vi "test prepared statement.vi"() -> ()   [LabVIEW 2020, in "mysql.lvlib" / "mysql.lvclass"]
uses:
  mysql.net/mysql.lvclass
panel:
  in  "Connection string":string="server=127.0.0.1;uid=root;pwd=Nitrog3n;database=test"
  in  "error in (no error)":errorcluster
  out "mysql out":refnum<class "mysql.lvclass">
  out "error out":errorcluster
  in  "Statement in":string
  in  "Parameters in":string[](array[string])
  out "Result":string[][](array[string])
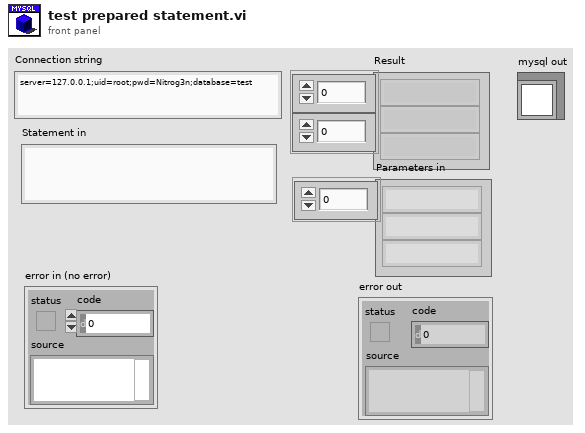
[diagram p1: front panel]
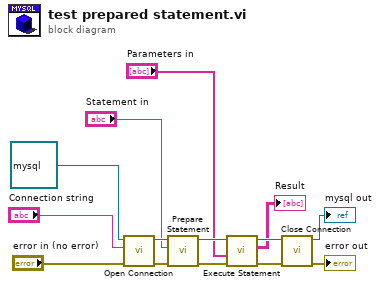
[diagram p0: block diagram]
diagram:
  n1 = call-dynamic "Open Connection.vi"("error in (no error)"="error in (no error)", "Connection string"="Connection string", "mysql in"=refnum<class "mysql.lvclass"> refnum) -> ("error out"=w13:errorcluster, "mysql out"=w14:refnum<class "mysql.lvclass">)  [unwired: 7 in]
  n2 = call-dynamic "Prepare Statement.vi"("error in (no error)"=w13, "Statement in"="Statement in", "mysql in"=w14) -> ("error out"=w11:errorcluster, "mysql out"=w12:refnum<class "mysql.lvclass">)  [unwired: 6 in, 1 out]
  n3 = call-dynamic "Execute Statement.vi"("error in (no error)"=w11, "Parameters in"="Parameters in", "mysql in"=w12) -> ("error out"=w9:errorcluster, "Result"=→"Result":string[][], "mysql out"=w10:refnum<class "mysql.lvclass">)  [unwired: 6 in]
  n4 = call-dynamic "Close Connection.vi"("error in (no error)"=w9, "mysql in"=w10) -> ("error out"=→"error out":errorcluster, "mysql out"=→"mysql out":refnum<class "mysql.lvclass">)  [unwired: 8 in]
